vi "Generate Service Config JSON_PostBuildActionCopy.vi"(0 "display name":string, 1 "description URL":string, 5 "service class":string, 7 "provided interfaces":string[](array[string]), 9 "path":string, 11 "error in":errorcluster, 12 "annotations":T1[](array[typedef])) -> (4 "service config JSON":string, 15 "error out":errorcluster)   [LabVIEW 2021]
uses:
  bc9aefa1-3362-4a2c-90c5-66f2f712a504.vi
  b5e8b0e6-3f85-492a-af2d-3d6fea27807d.vi
  66c50da6-e102-43cf-b33a-4f438f0b8493.vi
  5c69112c-150a-4d09-bff4-1bb7e67167f0.vi
  cf82bfed-f59b-4d13-8314-d7cde18762da.vi
  6b23a12b-55ed-4ced-adbb-94a3fce97b84.vi
  <vilib>/MeasurementLink/MeasurementLink Measurement Server/Helpers/TypeDefs/Measurement Annotation.ctl
  <vilib>/MeasurementLink/MeasurementLink Measurement Server/MeasurementLink Measurement Server.lvlib
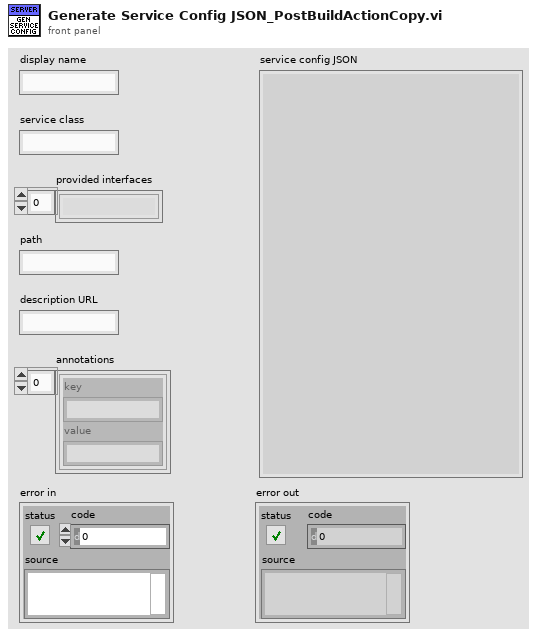
[diagram p1: front panel]
types:
  T1 = typedef "MeasurementLink Measurement Server.lvlib/Measurement Annotation.ctl" = cluster{"key":string, "value":string}
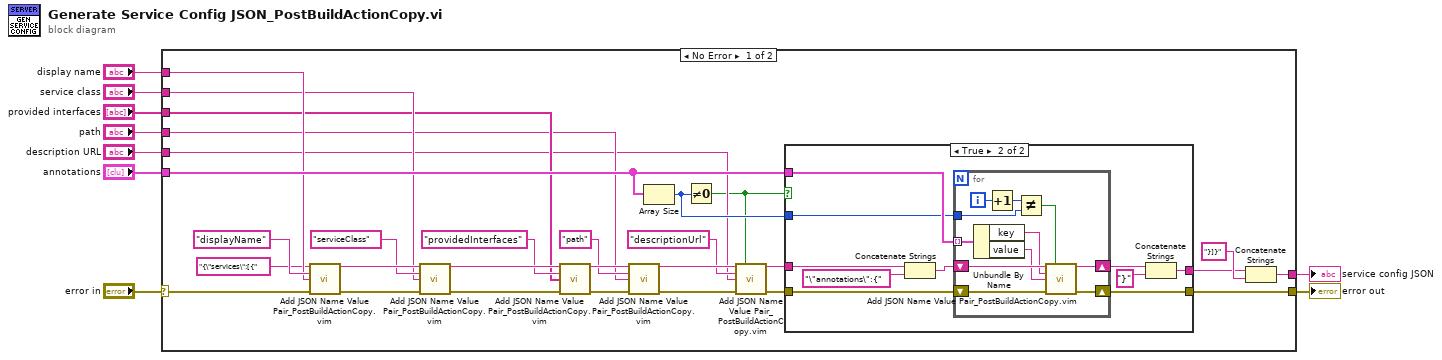
[diagram p0: block diagram]
diagram:
  n1 = case shown="No Error" "error in" {
    selector: "error in" -> [w32 w62]
    tunnel: [w36 w62] -> w8
    tunnel: "display name" -> [w30 _]
    tunnel: "service class" -> [w26 _]
    tunnel: "provided interfaces" -> [w22 _]
    tunnel: [w37 _] -> w4
    tunnel: "path" -> [w18 _]
    tunnel: "description URL" -> [w13 _]
    tunnel: "annotations" -> [w35 _]
    frame No Error {
      n2 = call "Add JSON Name Value Pair_PostBuildActionCopy.vim"("JSON string in"="{\"services\":[{", "name"="displayName", "value"=w30, "error in"=w32) -> ("JSON string out"=w28:string, "error out"=w29:errorcluster)  [unwired: 10 in]
      n3 = call "Add JSON Name Value Pair_PostBuildActionCopy.vim"("JSON string in"=w28, "name"="serviceClass", "value"=w26, "error in"=w29) -> ("JSON string out"=w24:string, "error out"=w25:errorcluster)  [unwired: 10 in]
      n4 = call "Add JSON Name Value Pair_PostBuildActionCopy.vim"("JSON string in"=w24, "name"="providedInterfaces", "value"=w22, "error in"=w25) -> ("JSON string out"=w20:string, "error out"=w21:errorcluster)  [unwired: 10 in]
      n5 = call "Add JSON Name Value Pair_PostBuildActionCopy.vim"("JSON string in"=w20, "name"="path", "value"=w18, "error in"=w21) -> ("JSON string out"=w15:string, "error out"=w17:errorcluster)  [unwired: 10 in]
      n6 = Array Size(array=w35) -> (size(s)=w34:i32)
      n7 = Not Equal To 0?(x=w34) -> (x != 0?=w12:bool)
      n8 = call "Add JSON Name Value Pair_PostBuildActionCopy.vim"("JSON string in"=w15, "include trailing comma"=w12, "name"="descriptionUrl", "value"=w13, "error in"=w17) -> ("JSON string out"=w11:string, "error out"=w16:errorcluster)  [unwired: 9 in]
      n9 = case shown="True" w12 {
        tunnel: w16 -> [w40 w50]
        tunnel: [w40 w49] -> w36
        tunnel: w35 -> [_ w48]
        tunnel: w34 -> [_ w45]
        tunnel: [w39 w42] -> w33
        tunnel: w11 -> [w39 w41]
        frame False {
        }
        frame True {
          n10 = Concatenate Strings(w41, "\"annotations\":{") -> (w46:string)
          n11 = for {
            shift-right: [w56] -> w49
            shift-left: w50 -> [w57]
            tunnel: w48 -> [w59] mode=indexing
            shift-right: [w54] -> w44
            shift-left: w46 -> [w55]
            tunnel: w45 -> [w58]
            i -> [w61]
            n12 = Unbundle By Name(w59) -> ("key"=w51:string, "value"=w52:string)
            n13 = Increment(x=w61) -> (x+1=w60:i32)
            n14 = Not Equal?(x=w60, y=w58) -> (x != y?=w53:bool)
            n15 = call "Add JSON Name Value Pair_PostBuildActionCopy.vim"("JSON string in"=w55, "include trailing comma"=w53, "name"=w51, "value"=w52, "error in"=w57) -> ("JSON string out"=w54:string, "error out"=w56:errorcluster)  [unwired: 9 in]
          }
          n16 = Concatenate Strings(w44, "}") -> (w42:string)
        }
      }
      n17 = Concatenate Strings(w33, "}]}") -> (w37:string)
    }
    frame Error {
    }
  }
  "error out" <- w8
  "service config JSON" <- w4
